vi "Open Actor ControlTerminal Ref.vi"(8 "error in (no error)":errorcluster, 10 "TopLevelDiagram in":refnum<vi>, 11 "ConPane":refnum<vi>) -> (0 "error out":errorcluster, 1 "Actor Input Found?":bool, 3 "Actor Input ControlTerminal":refnum<vi>)   [LabVIEW 2020, in "Add to Private Data.lvlib"]
uses:
  Add to Private Data.lvlib
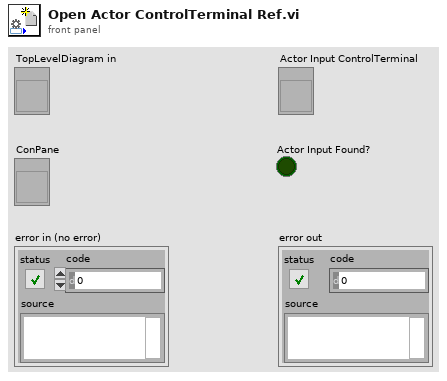
[diagram p1: front panel]
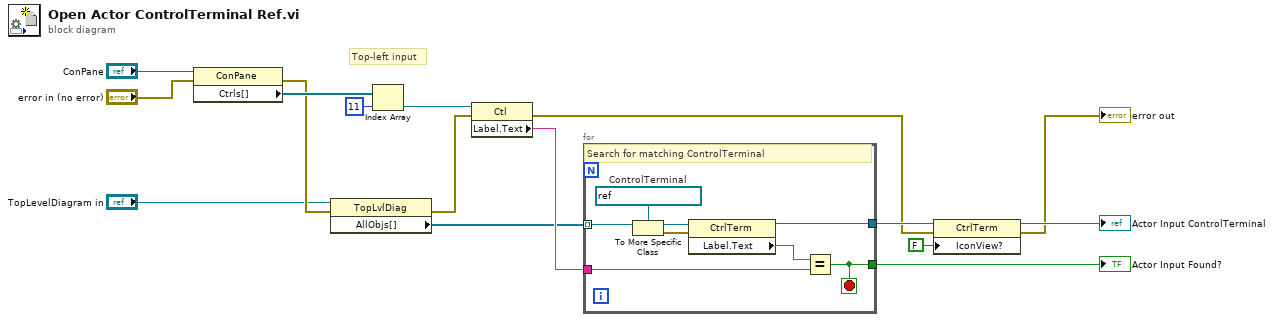
[diagram p0: block diagram]
diagram:
  # "Top-left input"
  n1 = property on="Property Node" class="ConPane"(reference="ConPane", error in="error in (no error)") -> (error out=w8:errorcluster, "Ctrls[]"=w11:refnum<vi>[])  [unwired: 1 out]
  n2 = property on="Property Node" class="TopLvlDiag"(reference="TopLevelDiagram in", error in=w8) -> (error out=w7:errorcluster, "AllObjs[]"=w14:refnum<vi>[])  [unwired: 1 out]
  n3 = Index Array(array=w11, index=11) -> (element=w13:refnum<vi>)
  n4 = property on="Property Node" class="Ctl"(reference=w13, error in=w7) -> (error out=w3:errorcluster, "Label.Text"=w15:string)  [unwired: 1 out]
  n5 = for {
    tunnel: w14 -> [w24] mode=indexing
    tunnel: w15 -> [w23]
    tunnel: [w18] -> w16
    tunnel: [w17] -> w6
    stop <- w17 stop-if-true
    w21 = refnum<vi> refnum  # ControlTerminal
    # "Search for matching ControlTerminal"
    n6 = To More Specific Class(target class=w21, reference=w24) -> (specific class reference=w22:refnum<vi>, error out=w20:errorcluster)  [unwired: 1 in]
    n7 = property class="CtrlTerm"(reference=w22, error in=w20) -> (reference out=w18:refnum<vi>, "Label.Text"=w19:string)  [unwired: 1 out]
    n8 = Equal?(x=w19, y=w23) -> (x = y?=w17:bool)
  }
  "Actor Input Found?" <- w6
  n9 = property class="CtrlTerm"(reference=w16, error in=w3, "IconView?"=FALSE ("Icon View?")) -> (reference out=→"Actor Input ControlTerminal":refnum<vi>, error out=→"error out":errorcluster)
